vi "Trilaterate.vi"(2 "C":cluster{"X":dbl, "Y":dbl, "Dist":dbl}, 3 "B":cluster{"X":dbl, "Y":dbl, "Dist":dbl}, 4 "A":cluster{"X":dbl, "Y":dbl, "Dist":dbl}) -> (0 "Y":dbl, 1 "X":dbl)   [LabVIEW 2015]
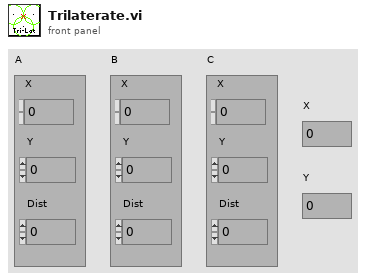
[diagram p1: front panel]
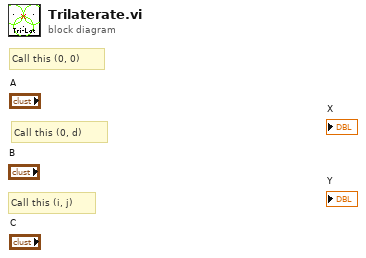
[diagram p0: block diagram]
diagram:
  # "Call this (i, j)"
  # "Call this (0, d)"
  # "Call this (0, 0)"
